vi "dataAcq_buffers_storage_reentrant.vi"(1 "interferogram prop set":T1 {"contrast" format="%.2f"; "OPDmax (cm)" format="%.2f"; "OPDmin (cm)" format="%.2f"; "peakToPeak position (cm)" format="%.2f"; "peakToPeak, (counts)" format="%.2f"; "X max (cm)" format="%.2f"; "X min (cm)" format="%.2f"}, 2 "action":T4(ring), 4 "spectrum prop set":T2 {"X max" format="%.2f"; "X min" format="%.2f"}, 6 "interferogram set":sgl[](array[numeric]) format="%.2f", 7 "spectrum set Y":sgl[](array[numeric]) format="%.2f", 9 "spectrum set X":sgl[](array[numeric]) format="%.2f") -> (11 "spectrum X":sgl[](array[numeric]) format="%.2f", 12 "interferogram":sgl[](array[numeric]) format="%.2f", 13 "spectrum Y":sgl[](array[numeric]) format="%.2f", 15 "interferogram prop":T1 {"contrast" format="%.2f"; "OPDmax (cm)" format="%.2f"; "OPDmin (cm)" format="%.2f"; "peakToPeak position (cm)" format="%.2f"; "peakToPeak, (counts)" format="%.2f"; "X max (cm)" format="%.2f"; "X min (cm)" format="%.2f"}, 18 "spectrum prop":T2 {"X max" format="%.2f"; "X min" format="%.2f"})   [LabVIEW 2010, in "OSA.lvclass"]
doc: "Latest retrieved data, (interferogram or spectrum), stored in this buffer vi."
uses:
  OSA.lvclass
  typeDef/spectrum_properties.ctl
  typeDef/xVal_option.ctl
  typeDef/interferogram_properties.ctl
panel:
  # "data per spectrometer \narranged in columns, (second index)"
  # "only Y data saved, (no X data created during sampling),\nto keep allocated data memory as small as possible."
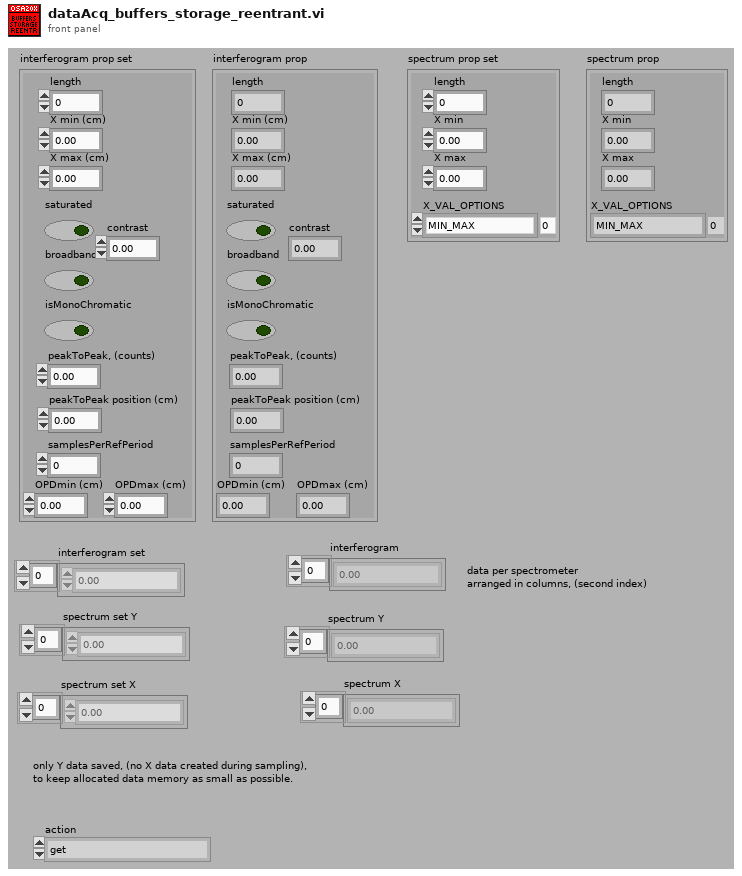
[diagram p1: front panel]
types:
  T1 = typedef "OSA.lvclass/interferogram_properties.ctl" = cluster{"length":u32, "X min (cm)":sgl, "X max (cm)":sgl, "saturated":bool, "broadband":bool, "isMonoChromatic":bool, "peakToPeak, (counts)":dbl, "peakToPeak position (cm)":dbl, "samplesPerRefPeriod":sgl, "OPDmin (cm)":sgl, "OPDmax (cm)":sgl, "contrast":dbl}
  T2 = typedef "OSA.lvclass/spectrum_properties.ctl" = cluster{"length":u32, "X min":sgl, "X max":sgl, "X_VAL_OPTIONS":T3}
  T3 = typedef "OSA.lvclass/xVal_option.ctl" = enum16{"MIN_MAX", "ARRAY"}
  T4 = enum16{"get", "init", "set interferogram", "set spectrum", "cleanUp"}
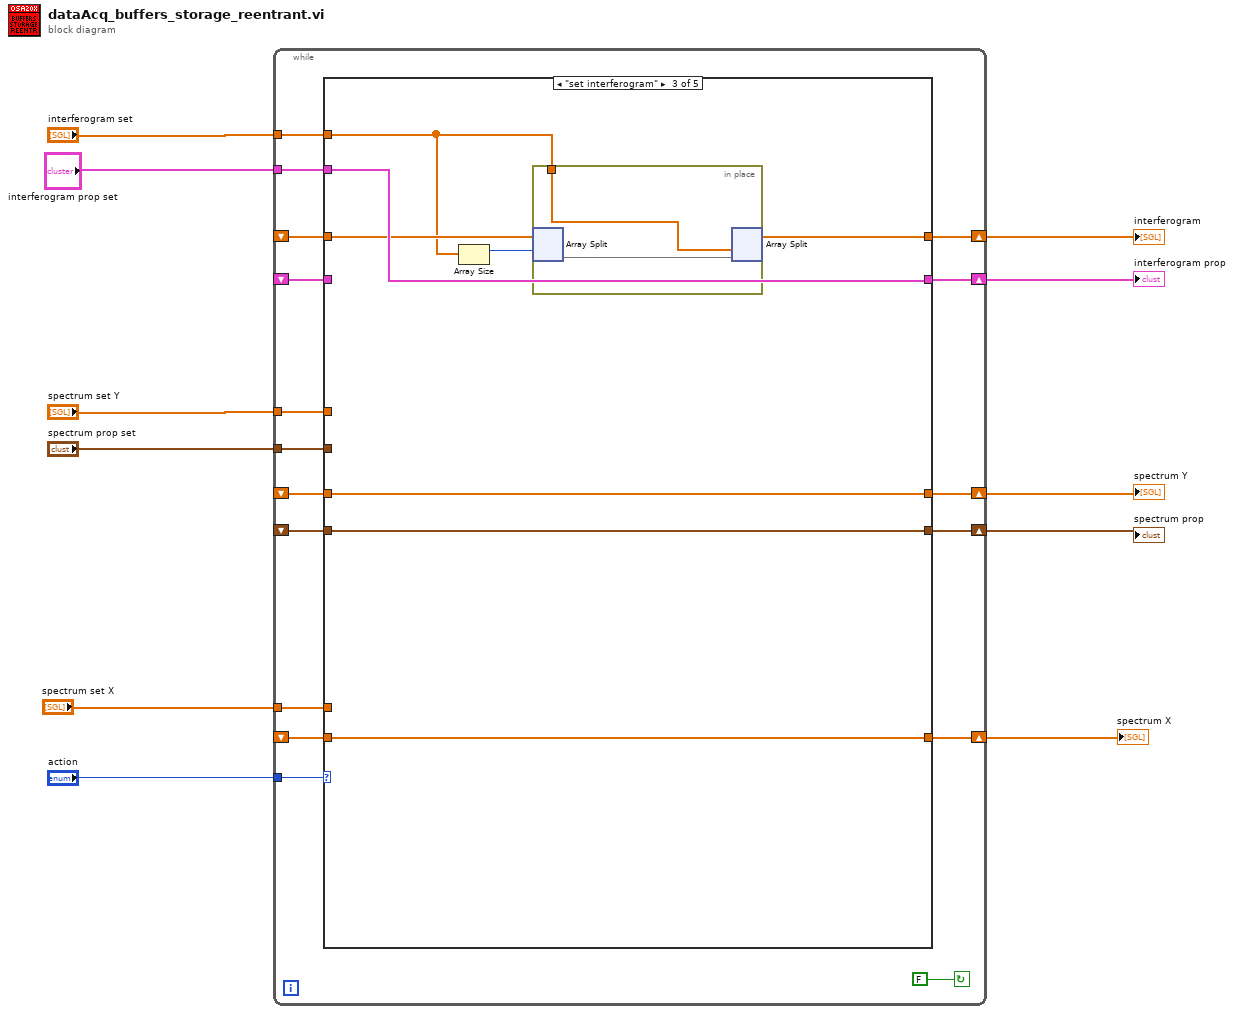
[diagram p0: block diagram]
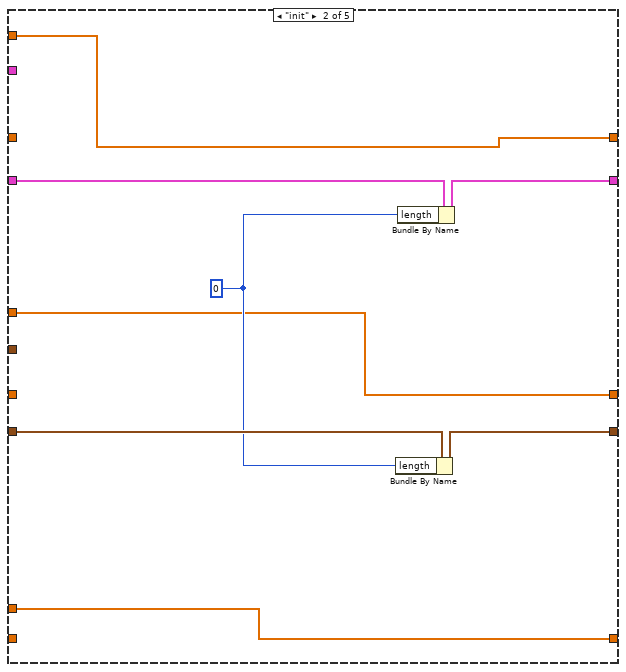
[diagram p3: hidden frame]
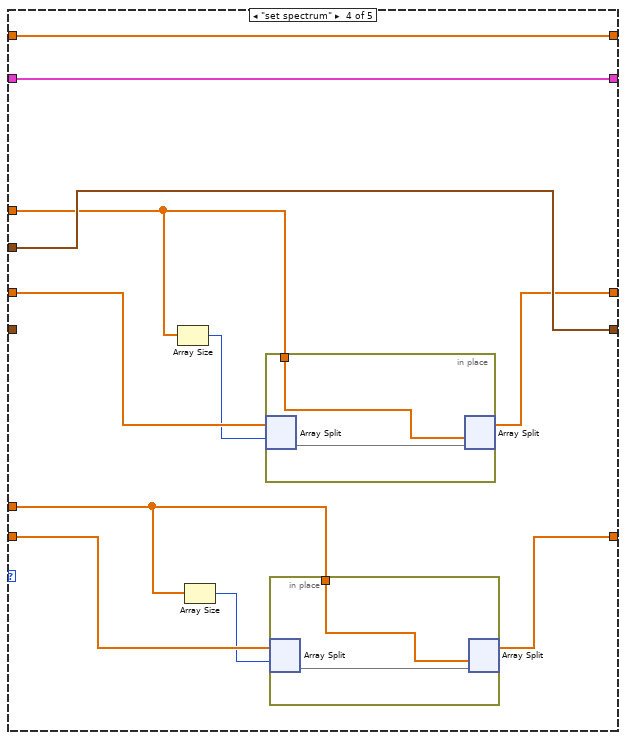
[diagram p4: hidden frame]
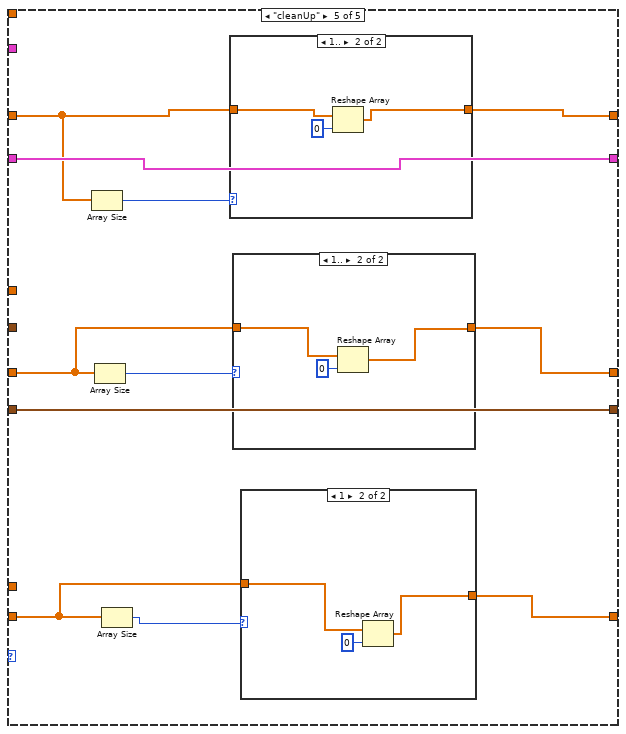
[diagram p5: hidden frame]
diagram:
  n1 = while {
    shift-right: [w25] -> w11
    shift-left: _ -> [w19]
    tunnel: "action" -> [w28]
    shift-right: [w24] -> w10
    shift-left: _ -> [w18]
    shift-right: [w23] -> w9
    shift-left: _ -> [w16]
    shift-right: [w21] -> w8
    shift-left: _ -> [w17]
    tunnel: "interferogram set" -> [w27]
    tunnel: "interferogram prop set" -> [w26]
    tunnel: "spectrum set Y" -> [w22]
    tunnel: "spectrum prop set" -> [w20]
    shift-right: [w13] -> w1
    shift-left: _ -> [w12]
    tunnel: "spectrum set X" -> [w14]
    stop <- FALSE continue-if-true
    n2 = case shown="\"set interferogram\"" w28 {
      tunnel: w27 -> [_ w36 w44 _ _]
      tunnel: w26 -> [_ _ w47 _ _]
      tunnel: [w33 w36 w43 w62 w74] -> w25
      tunnel: [w32 w38 w47 w61 w77] -> w24
      tunnel: [w30 w35 w49 w58 w73] -> w23
      tunnel: w22 -> [_ w35 _ w57 _]
      tunnel: [w31 w39 w48 w60 w76] -> w21
      tunnel: w20 -> [_ _ _ w60 _]
      tunnel: w19 -> [w33 _ w45 w62 w75]
      tunnel: w18 -> [w32 w41 _ w61 w77]
      tunnel: w17 -> [w31 w40 w48 _ w76]
      tunnel: w16 -> [w30 _ w49 w59 w70]
      tunnel: w14 -> [_ w34 _ w52 _]
      tunnel: [w29 w34 w42 w54 w67] -> w13
      tunnel: w12 -> [w29 _ w42 w56 w68]
      frame "get", Default {
      }
      frame "init" {
        w37 = u32 0 ("interferogram length set")
        n3 = Bundle By Name(cluster=w40, "length"=w37) -> (w39:T2)
        n4 = Bundle By Name(cluster=w41, "length"=w37) -> (w38:T1)
      }
      frame "set interferogram" {
        n5 = Array Size(array=w44) -> (size(s)=w46:i32)
        n6 = in-place {
          in-place-border: w44 -> [w51]
          n7 = in-place-split #1(w45, w46) -> (w50:sgl[])  [unwired: 1 out]
          n8 = in-place-split #1(w51, w50) -> (w43:sgl[])  [unwired: 1 out]
        }
      }
      frame "set spectrum" {
        n9 = Array Size(array=w57) -> (size(s)=w55:i32)
        n10 = Array Size(array=w52) -> (size(s)=w53:i32)
        n11 = in-place {
          in-place-border: w57 -> [w66]
          n12 = in-place-split #2(w59, w55) -> (w65:sgl[])  [unwired: 1 out]
          n13 = in-place-split #2(w66, w65) -> (w58:sgl[])  [unwired: 1 out]
        }
        n14 = in-place {
          in-place-border: w52 -> [w64]
          n15 = in-place-split #3(w56, w53) -> (w63:sgl[])  [unwired: 1 out]
          n16 = in-place-split #3(w64, w63) -> (w54:sgl[])  [unwired: 1 out]
        }
      }
      frame "cleanUp" {
        n17 = Array Size(array=w75) -> (size(s)=w72:i32)
        n18 = Array Size(array=w70) -> (size(s)=w71:i32)
        n19 = Array Size(array=w68) -> (size(s)=w69:i32)
        n20 = case shown="1.." w72 {
          tunnel: w75 -> [w86 w89]
          tunnel: [w86 w88] -> w74
          frame 0, Default {
          }
          frame 1.. {
            n21 = Reshape Array(w89, 0 ("dimension size")) -> (w88:sgl[])
          }
        }
        n22 = case shown="1.." w71 {
          tunnel: w70 -> [w82 w85]
          tunnel: [w82 w84] -> w73
          frame 0, Default {
          }
          frame 1.. {
            n23 = Reshape Array(w85, 0 ("dimension size")) -> (w84:sgl[])
          }
        }
        n24 = case shown="1" w69 {
          tunnel: w68 -> [w78 w80]
          tunnel: [w78 w79] -> w67
          frame 0, Default {
          }
          frame 1 {
            n25 = Reshape Array(w80, 0 ("dimension size")) -> (w79:sgl[])
          }
        }
      }
    }
  }
  "interferogram" <- w11
  "interferogram prop" <- w10
  "spectrum Y" <- w9
  "spectrum prop" <- w8
  "spectrum X" <- w1
